vi "CLD 11 CSV file utility.vi"(8 "Fehler (Eingang)":T1, 10 "[Daten, Eingang]":T2[](array[typedef]), 11 "CSV-Datei-Enum":T3) -> (0 "Fehler (Ausgang)":T1, 3 "[Daten, Ausgang]":T2[](array[typedef]))   [LabVIEW 2009]
doc: "CLD 11 - Datei-Utility aus CLD 6"
uses:
  <vilib>/Utility/file.llb/Read From Spreadsheet File (string).vi
  CLD 11 CSV file data structure.ctl
  <vilib>/Utility/file.llb/Write To Spreadsheet File (string).vi
  CLD 11 CSV file enum.ctl
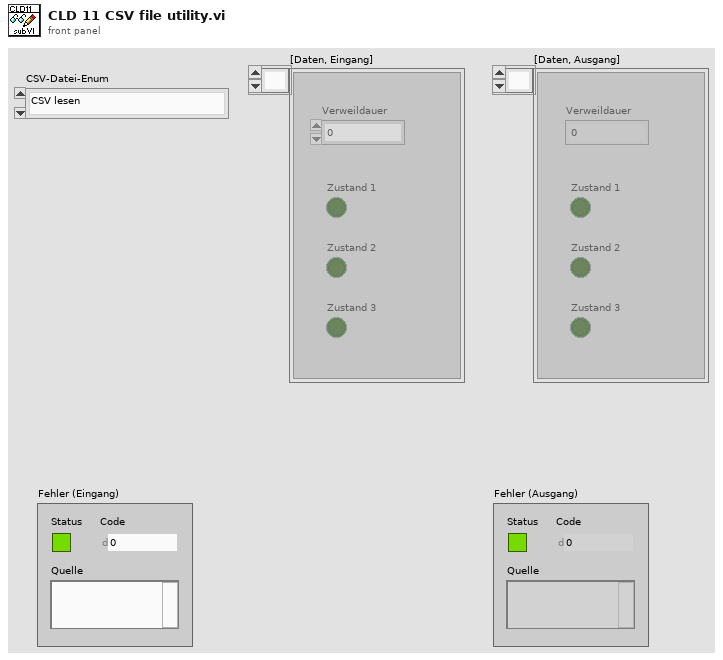
[diagram p1: front panel]
types:
  T1 = cluster{"Status":bool, "Code":i32, "Quelle":string}
  T2 = typedef "CLD 11 CSV file data structure.ctl" = cluster{"Verweildauer":i32, "Zustand 1":bool, "Zustand 2":bool, "Zustand 3":bool}
  T3 = typedef "CLD 11 CSV file enum.ctl" = enum16{"CSV lesen", "CSV schreiben"}
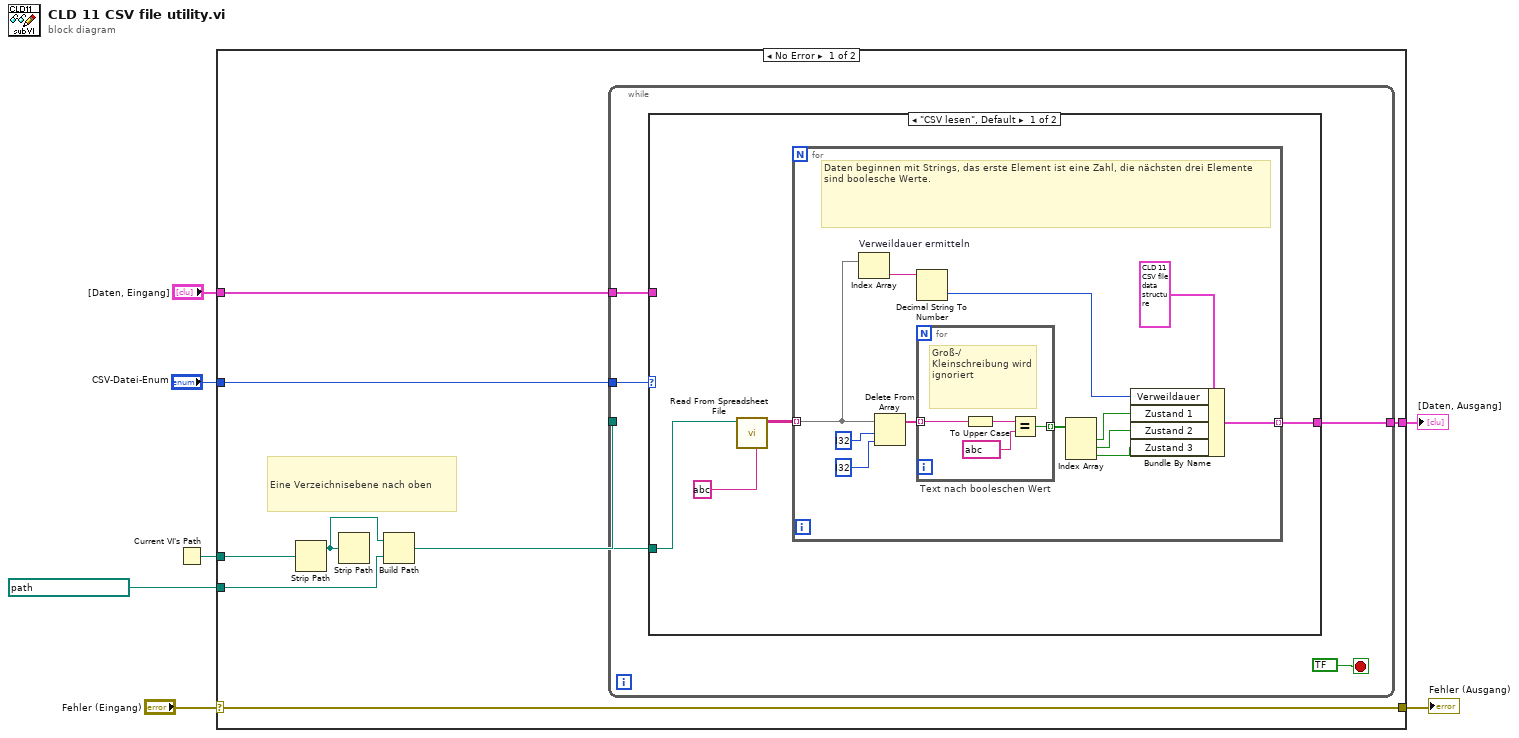
[diagram p0: block diagram]
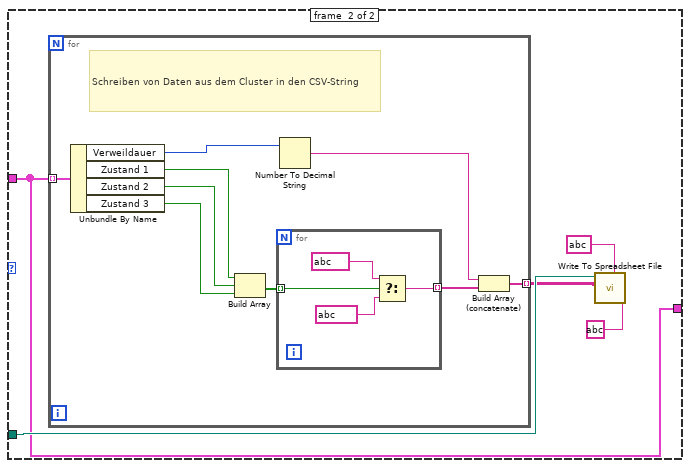
[diagram p2: hidden frame]
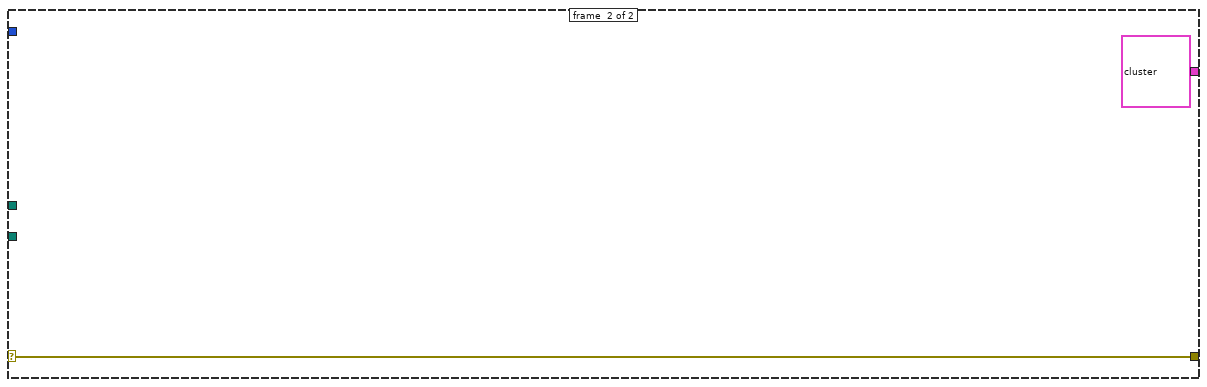
[diagram p3: hidden frame]
diagram:
  n1 = Current VI's Path() -> (path=w5:path)
  n2 = case shown="No Error" "Fehler (Eingang)" {
    selector: "Fehler (Eingang)" -> [w9 w60]
    tunnel: [w15 T2[] ? ("[Daten, Eingang]")] -> w7
    tunnel: path ? -> [w14 _]
    tunnel: w5 -> [w13 _]
    tunnel: "CSV-Datei-Enum" -> [w11 _]
    tunnel: "[Daten, Eingang]" -> [w10 _]
    tunnel: [w9 w60] -> w1
    frame #0 {
      # "Eine Verzeichnisebene nach oben"
      n3 = Strip Path(path=w13) -> (stripped path=w8:path)  [unwired: 1 out]
      n4 = Strip Path(path=w8) -> ()  [unwired: 2 out]
      n5 = Build Path(base path=w8, name or relative path=w14) -> (appended path=w12:path)
      n6 = while {
        tunnel: w12 -> [w18]
        tunnel: w11 -> [w19]
        tunnel: [w17] -> w15
        tunnel: w10 -> [w16]
        stop <- bool ? stop-if-true
        n7 = case shown="\"CSV lesen\", Default" w19 {
          tunnel: w18 -> [w24 w45]
          tunnel: [w22 w41] -> w17
          tunnel: w16 -> [_ w41]
          frame #0 {
            n8 = call-poly <vilib>:"Read From Spreadsheet File.vi"("delimiter (\\t)"=string ? ("Trennzeichen (\\t)"), "file path (dialog if empty)"=w24) -> ("all rows"=w23:string[][])  [unwired: 5 in, 4 out]
            n9 = for {
              tunnel: w23 -> [w33] mode=indexing
              tunnel: [w36] -> w22 mode=indexing
              # "Daten beginnen mit Strings, das erste Element ist eine Zahl, die nächsten drei Elemente sind boolesche Werte."
              n10 = Index Array "Verweildauer ermitteln"(array=w33) -> (element=w35:string)  [unwired: 1 in]
              n11 = Delete From Array(array=w33, length=i32 ? ("Länge"), index=i32 ? ("Index")) -> (array with subset deleted=w26:string[])  [unwired: 1 out]
              n12 = Decimal String To Number(string=w35) -> (number=w34:i32)  [unwired: 2 in, 1 out]
              n13 = for "Text nach booleschen Wert" {
                tunnel: w26 -> [w40] mode=indexing
                tunnel: [w37] -> w30 mode=indexing
                # "Groß-/Kleinschreibung wird ignoriert"
                n14 = To Upper Case(1:w40) -> (0:w39:string)
                n15 = Equal?(x=w39, y=string ?) -> (x = y?=w37:bool)
              }
              n16 = Index Array(array=w30) -> (element #1=w29:bool, element #2=w28:bool, element #3=w27:bool)  [unwired: 3 in]
              n17 = Bundle By Name(cluster=T2 ? ("Datenstruktur der CSV-Datei"), "Verweildauer"=w34, "Zustand 1"=w29, "Zustand 2"=w28, "Zustand 3"=w27) -> (w36:T2)
            }
          }
          frame #1 {
            n18 = for {
              tunnel: w41 -> [w54] mode=indexing
              tunnel: [w46] -> w43 mode=indexing
              # "Schreiben von Daten aus dem Cluster in den CSV-String"
              n19 = Unbundle By Name(w54) -> ("Verweildauer"=w53:i32, "Zustand 1"=w52:bool, "Zustand 2"=w51:bool, "Zustand 3"=w50:bool)
              n20 = Build Array(w52, w51, w50) -> (w49:bool[])
              n21 = for {
                tunnel: w49 -> [w58] mode=indexing
                tunnel: [w55] -> w47 mode=indexing
                n22 = Select(t=string ?, s=w58, f=string ?) -> (s? t:f=w55:string)
              }
              n23 = Number To Decimal String(number=w53) -> (decimal integer string=w48:string)  [unwired: 1 in]
              n24 = Build Array (concatenate)(w48, w47) -> (w46:string[])
            }
            n25 = call-poly <vilib>:"Write To Spreadsheet File.vi"("delimiter (\\t)"=string ? ("Trennzeichen (\\t)"), "format (%s)"=string ? ("Format (%s)"), "2D data"=w43, "file path (dialog if empty)"=w45) -> ()  [unwired: 4 in, 1 out]
          }
        }
      }
    }
    frame #1 {
    }
  }
  "[Daten, Ausgang]" <- w7
  "Fehler (Ausgang)" <- w1
